vi "Example - DataType float.vi"() -> ()   [LabVIEW 2017]
uses:
  63d4ee60-3d36-44f6-9846-d3c89712fa4e.vi
  5d5e870e-b8ec-4111-8fcd-715cbb1e366c.vi
  6ca2ea0b-5a64-4cad-9736-18ec21bbeae0.vi
  4ee676fc-47c0-4be0-9ff8-88677d132e6f.vi
  a152669e-7808-472e-ac68-82058263c032.vi
  API-String-Arugments-Support/_Support/Data To API String Arguments.vi
  API-String-Arugments-Support/_Support/Convert API String Arguments to Data(variant).vi
panel:
  out "Array 3":T1(array[cluster]) {"Data" format="%#_6e"}
  out "concatenated string":string
  out "Array 2":T2(array[cluster]) {"?" format="%#_6e"; "Data" format="%#_6e"}
  out "Array":T2(array[cluster]) {"?" format="%#_6e"; "Data" format="%#_6e"}
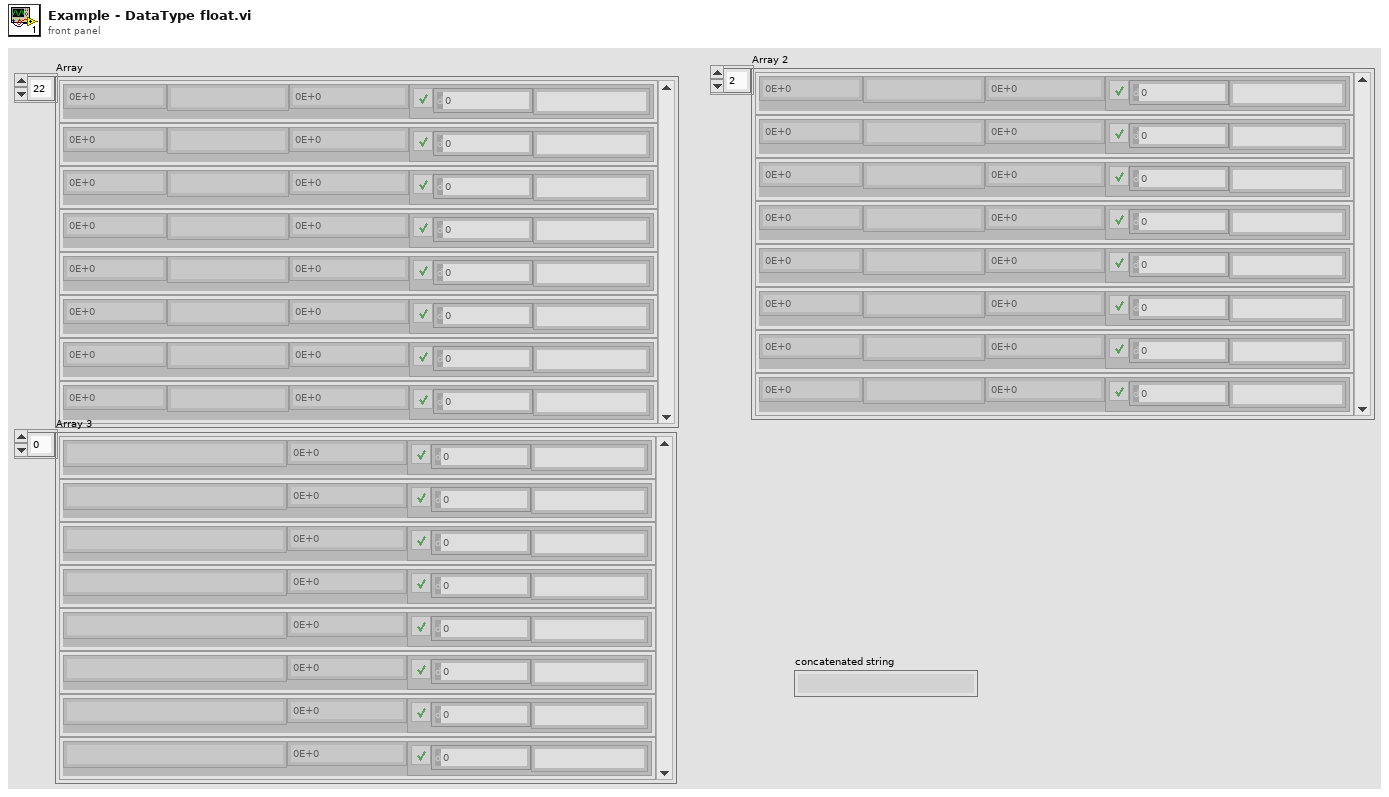
[diagram p1: front panel]
types:
  T1 = cluster{"String":string, "Data":dbl, "error":errorcluster}[]
  T2 = cluster{dbl, "String":string, "Data":dbl, "error":errorcluster}[]
  T3 = cluster{dbl, "String":string, "Data":dbl, "error":errorcluster}
  T4 = cluster{"string":string, "Data":dbl, "error":errorcluster}
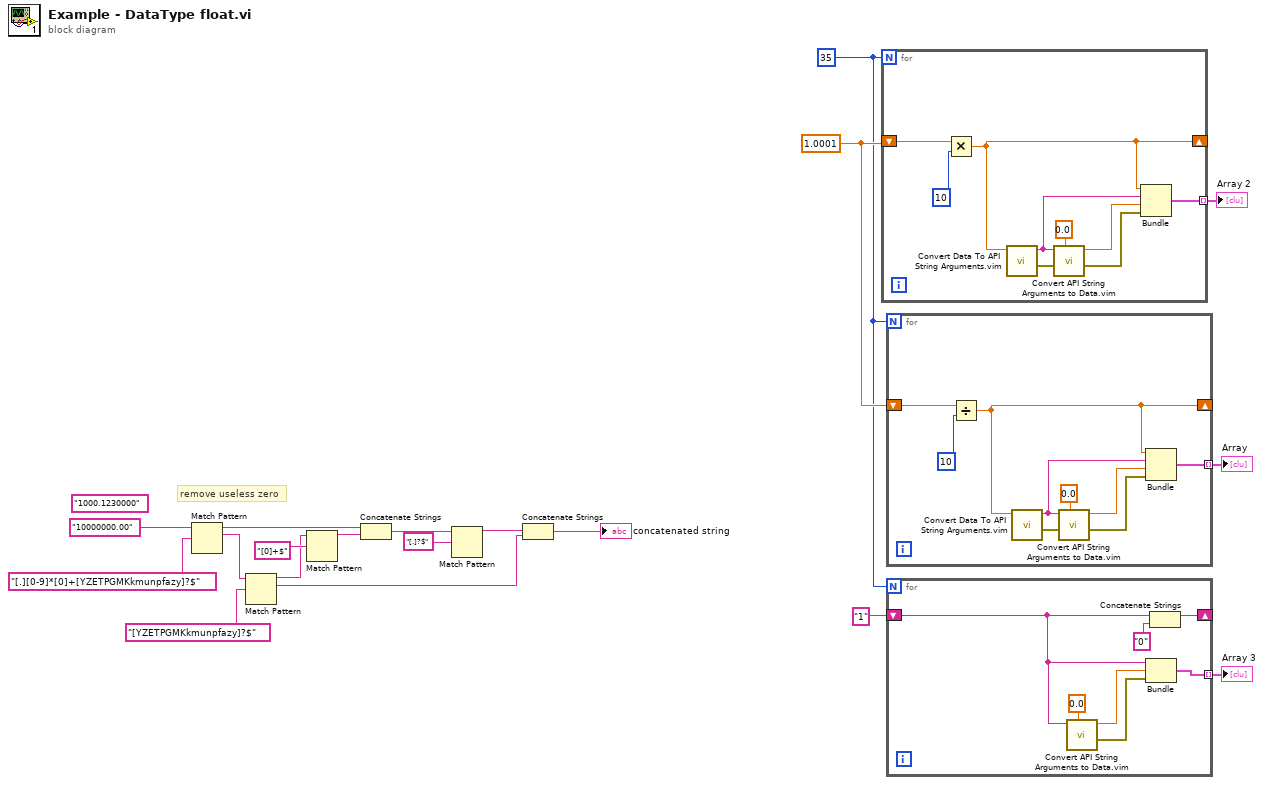
[diagram p0: block diagram]
diagram:
  (unwired) "1000.1230000" ("string")
  w13 = 1.0001
  w11 = 35
  # "remove useless zero"
  n1 = Match Pattern(string="10000000.00", regular expression="[.][0-9]*[0]+[YZETPGMKkmunpfazy]?$") -> (before substring=w16:string, match substring=w8:string)  [unwired: 1 in, 2 out]
  n2 = Match Pattern(string=w8, regular expression="[YZETPGMKkmunpfazy]?$") -> (before substring=w6:string, match substring=w2:string)  [unwired: 1 in, 2 out]
  n3 = Match Pattern(string=w6, regular expression="[0]+$") -> (before substring=w7:string)  [unwired: 1 in, 3 out]
  n4 = Concatenate Strings(w16, w7) -> (w4:string)
  n5 = Match Pattern(string=w4, regular expression="[.]?$") -> (before substring=w3:string)  [unwired: 1 in, 3 out]
  n6 = Concatenate Strings(w3, w2) -> (→"concatenated string":string)
  n7 = for {
    N: w11 -> [_]
    shift-right: [w24] -> _
    shift-left: w13 -> [w27]
    tunnel: [w20] -> w18 mode=indexing
    n8 = Multiply(x=w27, y=10) -> (x*y=w24:dbl)
    n9 = call "Convert Data To API String Arguments.vim"("data"=w24) -> ("error out"=w25:errorcluster, "String"=w23:string)  [unwired: 7 in]
    n10 = call "Convert API String Arguments to Data.vim"("Type"=0.0, "error in (no error)"=w25, "String"=w23) -> ("error"=w21:errorcluster, "Data"=w22:dbl)  [unwired: 5 in]
    n11 = Bundle(w24, "String"=w23, "Data"=w22, "error"=w21) -> (w20:T3)  [unwired: 1 in]
  }
  "Array 2" <- w18
  n12 = for {
    N: w11 -> [_]
    shift-right: [w33] -> _
    shift-left: w13 -> [w36]
    tunnel: [w29] -> w19 mode=indexing
    n13 = Divide(x=w36, y=10) -> (x/y=w33:dbl)
    n14 = call "Convert Data To API String Arguments.vim"("data"=w33) -> ("error out"=w34:errorcluster, "String"=w32:string)  [unwired: 7 in]
    n15 = call "Convert API String Arguments to Data.vim"("Type"=0.0, "error in (no error)"=w34, "String"=w32) -> ("error"=w30:errorcluster, "Data"=w31:dbl)  [unwired: 5 in]
    n16 = Bundle(w33, "String"=w32, "Data"=w31, "error"=w30) -> (w29:T3)  [unwired: 1 in]
  }
  "Array" <- w19
  n17 = for {
    N: w11 -> [_]
    shift-right: [w40] -> _
    shift-left: "1" ("string") -> [w38]
    tunnel: [w41] -> w12 mode=indexing
    n18 = call "Convert API String Arguments to Data.vim"("Type"=0.0, "String"=w38) -> ("error"=w42:errorcluster, "Data"=w43:dbl)  [unwired: 6 in]
    n19 = Bundle("string"=w38, "Data"=w43, "error"=w42) -> (w41:T4)  [unwired: 1 in]
    n20 = Concatenate Strings(w38, "0" ("string")) -> (w40:string)
  }
  "Array 3" <- w12
